vi "Finish.vi"   [LabVIEW 2017]
doc: "This VI is called during exit. It can be used to close I/O refnums, save collected data, etc."
uses:
  <vilib>/Rock Robotics/WPI/Utilities/WPI_GetSetVariantRefNum.vi
types:
  T1 = typedef "WPI_JoystickDevRef.ctl" = cluster{"Device":T2}
  T2 = typedef "WPI_JoystickDeviceEnum.ctl" = enum16{"USB 0", "USB 1", "USB 2", "USB 3", "USB 4", "USB 5"}
  T3 = typedef "WPI_SwitchDevRef.ctl" = cluster{"DevStatus":errorcluster, "DIO Channel":T4, "CntIndex":T5, "Normally Closed":bool}
  T4 = typedef "FPGA_DIOChannel.ctl" = enum8{"DIO 0", "DIO 1", "DIO 2", "DIO 3", "DIO 4", "DIO 5", "DIO 6", "DIO 7", "DIO 8", "DIO 9", "DIO MXP 0", "DIO MXP 1", "DIO MXP 2", "DIO MXP 3", "DIO MXP 4", "DIO MXP 5", "DIO MXP 6", "DIO MXP 7", "DIO MXP 8", "DIO MXP 9", "DIO MXP 10", "DIO MXP 11", "DIO MXP 12", "DIO MXP 13", "DIO MXP 14", "DIO MXP 15", "SPI Port CS1", "SPI Port CS2", "SPI Port CS3", "SPI Port MISO", "SPI Port MOSI", "Invalid"}
  T5 = typedef "FPGA_CounterCtrSystemIndex.ctl" = enum8{"Ctr 0", "Ctr 1", "Ctr 2", "Ctr 3", "Ctr 4", "Ctr 5", "Ctr 6", "Ctr 7", "Invalid"}
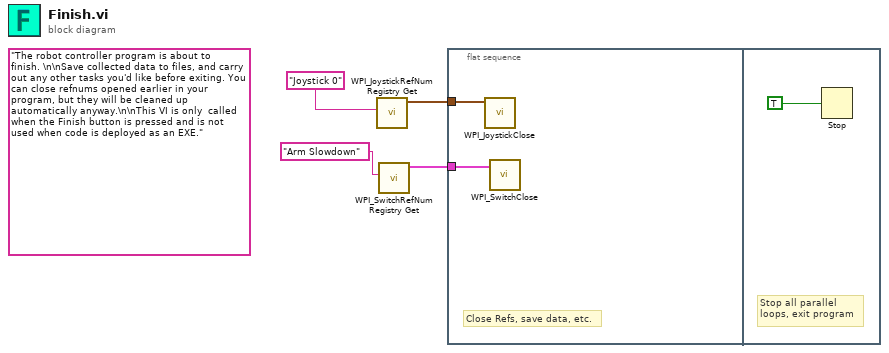
[diagram p0: block diagram]
diagram:
  (unwired) "The robot controller program is about to finish. \n\nSave collected data to files, and carry out any other tasks you'd like before exiting. You can close refnums opened earlier in your program, but they will be cleaned up automatically anyway.\n\nThis VI is only  called when the Finish button is pressed and is not used when code is deployed as an EXE."
  n1 = call <vilib>:"WPI_JoystickRefNum Registry Get.vi"("refnum name"="Joystick 0") -> ("JoystickDevRef"=w3:T1)  [unwired: 1 in, 9 out]
  n2 = call <vilib>:"WPI_SwitchRefNum Registry Get.vi"("refnum name"="Arm Slowdown") -> ("SwitchDevRef"=w1:T3)  [unwired: 9 in, 1 out]
  n3 = flat-sequence {
    tunnel: w3 -> [w6]
    tunnel: w1 -> [w5]
    frame #0 {
      # "Close Refs, save data, etc."
      n4 = call <vilib>:"WPI_JoystickClose.vi"("JoystickDevRef"=w6) -> ()  [unwired: 11 out]
      n5 = call <vilib>:"WPI_SwitchClose.vi"("SwitchDevRef"=w5) -> ()  [unwired: 10 in, 1 out]
    }
    frame #1 {
      # "Stop all parallel\nloops, exit program"
      n6 = Stop(stop? (T)=TRUE ("Quit")) -> ()
    }
  }
